vi "Init.vi"(11 "Refs":T4) -> (3 "Loop data init":T1)   [LabVIEW 2021, in "TipStripOOPanel.lvlib"]
uses:
  TipStripOOPanel.lvlib
  refs.ctl
  Loop Data Parent.ctl
  <vilib>/IlluminatedG/IG OOPanel/OOPanel/Manager/Manager.lvclass
  Classes/TipPanel/TipPanel.lvclass
  PanelMap.ctl
  PanelMapData.ctl
  Classes/TipPanel/ToPanelUEWrapper.ctl
  Classes/TipPanel/ToPanelUE.ctl
  <vilib>/Futures/Futures/Promise/Promise.lvclass
  <vilib>/Utility/miscctls.llb/LVRectTypeDef.ctl
  <vilib>/Utility/miscctls.llb/LVBoundsTypeDef.ctl
  <vilib>/Utility/miscctls.llb/LVPointTypeDef.ctl
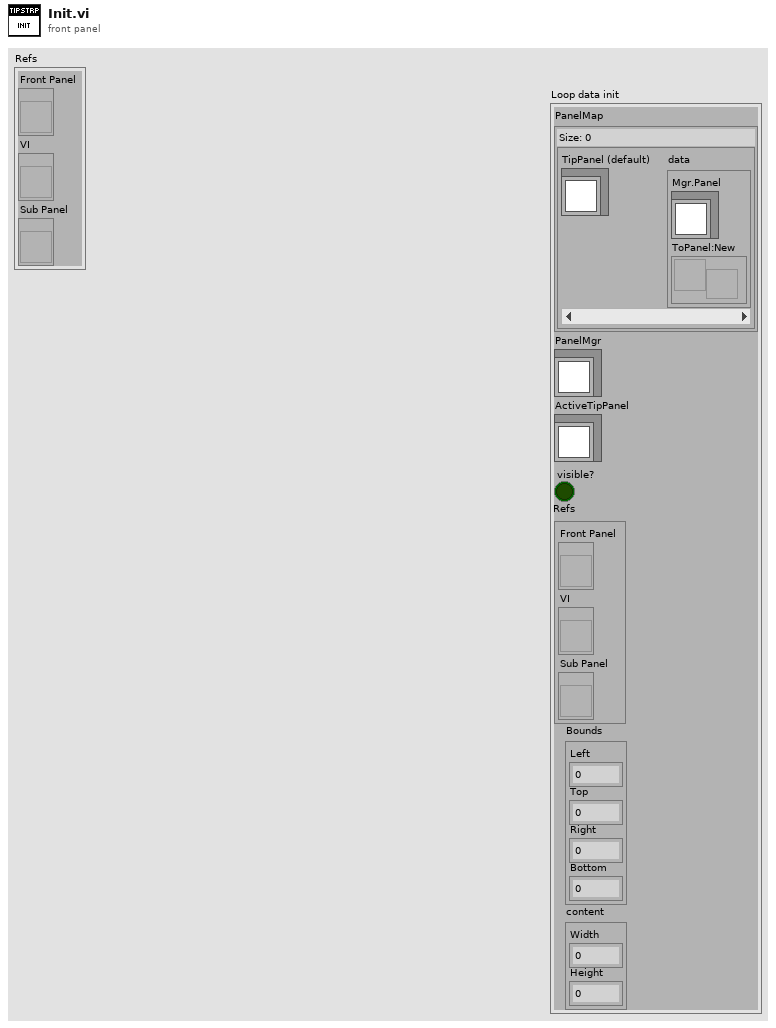
[diagram p1: front panel]
types:
  T1 = typedef "TipStripOOPanel.lvlib/Loop Data Parent.ctl" = cluster{"PanelMap":T2, "PanelMgr":refnum<class "Manager.lvclass">, "ActiveTipPanel":refnum<class "TipPanel.lvclass">, "visible?":bool, "Refs":T4, "Bounds":T5, "content":T6}
  T2 = typedef "TipStripOOPanel.lvlib/PanelMap.ctl" = map{refnum<class "TipPanel.lvclass">, T3}
  T3 = typedef "TipStripOOPanel.lvlib/PanelMapData.ctl" = cluster{"Mgr.Panel":refnum<class "TipPanel.lvclass">, "ToPanel:New":refnum<user-event>}
  T4 = typedef "TipStripOOPanel.lvlib/refs.ctl" = cluster{"Front Panel":refnum<vi>, "VI":refnum<vi>, "Sub Panel":refnum<vi>}
  T5 = typedef "LVRectTypeDef.ctl" = cluster{"Left":i16, "Top":i16, "Right":i16, "Bottom":i16}
  T6 = typedef "LVBoundsTypeDef.ctl" = cluster{"Width":u32, "Height":u32}
  T7 = typedef "LVPointTypeDef.ctl" = cluster{"Horizontal":i16, "Vertical":i16}
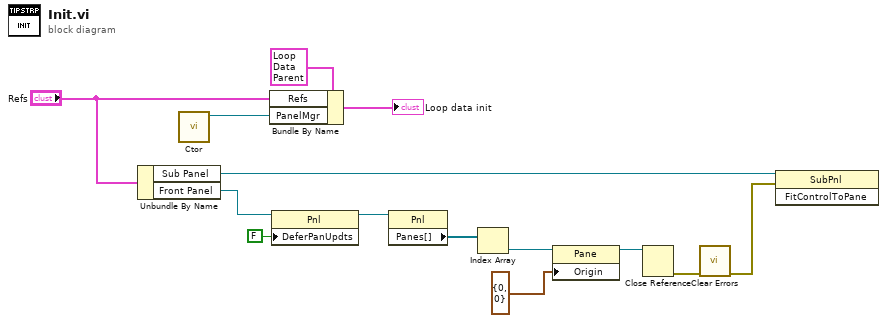
[diagram p0: block diagram]
diagram:
  n1 = Unbundle By Name("Refs") -> ("Sub Panel"=w10:refnum<vi>, "Front Panel"=w9:refnum<vi>)
  n2 = call <vilib>:"Ctor.vi"() -> ("Manager out"=w13:refnum<class "Manager.lvclass">)  [unwired: 10 in, 1 out]
  n3 = Bundle By Name(cluster=T1 {"PanelMap"={}, "PanelMgr"=refnum, "ActiveTipPanel"=refnum, "visible?"=FALSE, "Refs"={"Front Panel"=refnum, "VI"=refnum, "Sub Panel"=refnum}, "Bounds"={"Left"=0, "Top"=0, "Right"=0, "Bottom"=0}, "content"={"Width"=0, "Height"=0}} ("Cluster"), "Refs"="Refs", "PanelMgr"=w13) -> (→"Loop data init":T1)
  n4 = property class="Pnl"(reference=w9, "DeferPanUpdts"=FALSE ("Defer Panel Updates")) -> (reference out=w7:refnum<vi>)  [unwired: 1 in, 1 out]
  n5 = property class="Pnl"(reference=w7) -> ("Panes[]"=w6:refnum<vi>[])  [unwired: 1 in, 2 out]
  n6 = Index Array(array=w6) -> (element=w5:refnum<vi>)  [unwired: 1 in]
  n7 = property class="Pane"(reference=w5, "Origin"=T7 {"Horizontal"=0, "Vertical"=0}) -> (reference out=w3:refnum<vi>)  [unwired: 1 in, 1 out]
  n8 = Close Reference(reference=w3) -> (error out=w2:errorcluster)  [unwired: 1 in]
  n9 = call <vilib>:"Clear Errors.vi"("error in (no error)"=w2) -> ("error out"=w1:errorcluster)  [unwired: 5 in, 1 out]
  n10 = invoke class="SubPnl" method="FitControlToPane"(reference=w10, error in=w1) -> ()  [unwired: 1 in, 3 out]
